vi "LVClass_Pupil Write Pupil.vi"(8 "error in (no error)":errorcluster, 10 "Pupil":i32, 11 "Pupil in":refnum<class "Pupil.lvclass">) -> (0 "error out":errorcluster, 3 "Pupil out":refnum<class "Pupil.lvclass">)   [LabVIEW 2020, in "Pupil.lvclass"]
uses:
  Pupil.lvclass
  Handle creation.ctl
  Pupil.lvclass/Pupil.ctl
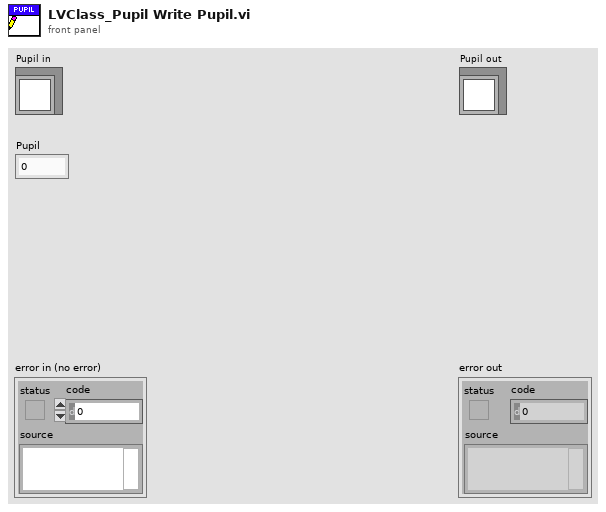
[diagram p1: front panel]
types:
  T1 = typedef "Handle creation.ctl" = enum16{"By ctor", "By write function"}
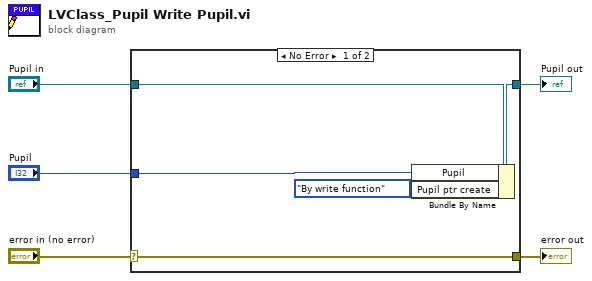
[diagram p0: block diagram]
diagram:
  n1 = case shown="No Error" "error in (no error)" {
    selector: "error in (no error)" -> [w10 w11]
    tunnel: [w10 w11] -> w4
    tunnel: [w8 w12] -> w2
    tunnel: "Pupil in" -> [w9 w12]
    tunnel: "Pupil" -> [w7 _]
    frame No Error {
      n2 = Bundle By Name(cluster=w9, "Pupil"=w7, "Pupil ptr create"=Handle_creation."By write function") -> (w8:refnum<class "Pupil.lvclass">)
    }
    frame Error {
    }
  }
  "error out" <- w4
  "Pupil out" <- w2
